vi "EXO1_DatabaseWrite_valves.vi"() -> ()   [LabVIEW 2012]
uses:
  <vilib>/addons/database/Connection.llb/DB Tools Open Connec (Path).vi
  <vilib>/addons/database/NI_Database_API.lvlib
panel:
  in  "V-15":bool
  in  "V-14":bool
  in  "V-13":bool
  in  "V-12":bool
  in  "V-11":bool
  in  "V-10":bool
  in  "V-9":bool
  in  "V-8":bool
  in  "V-7":bool
  in  "V-6":bool
  in  "V-5":bool
  in  "V-4":bool
  in  "V-3":bool
  in  "V-2":bool
  in  "V-1":bool
  in  "stop":bool
  out "current time":timestamp
  in  "Table Name (The table that you want to save the data into)":string="EXOvalve"
  # "EXO DatabaseWrite Sub-VI (II)"
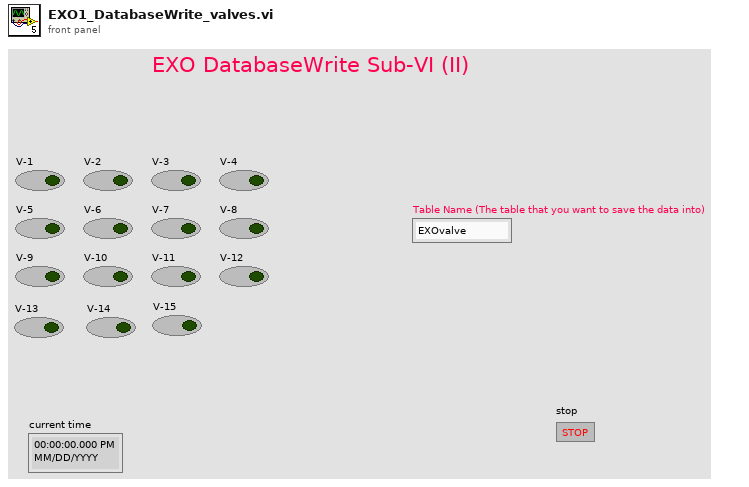
[diagram p1: front panel]
types:
  T1 = typedef "NI_Database_API.lvlib/Conn ObjectReference.ctl" = refnum<k1>
  T2 = cluster{dbl, "date/time string":string, string, string, string, string, string, string, string, string, string, string, string, string, string, string, string}
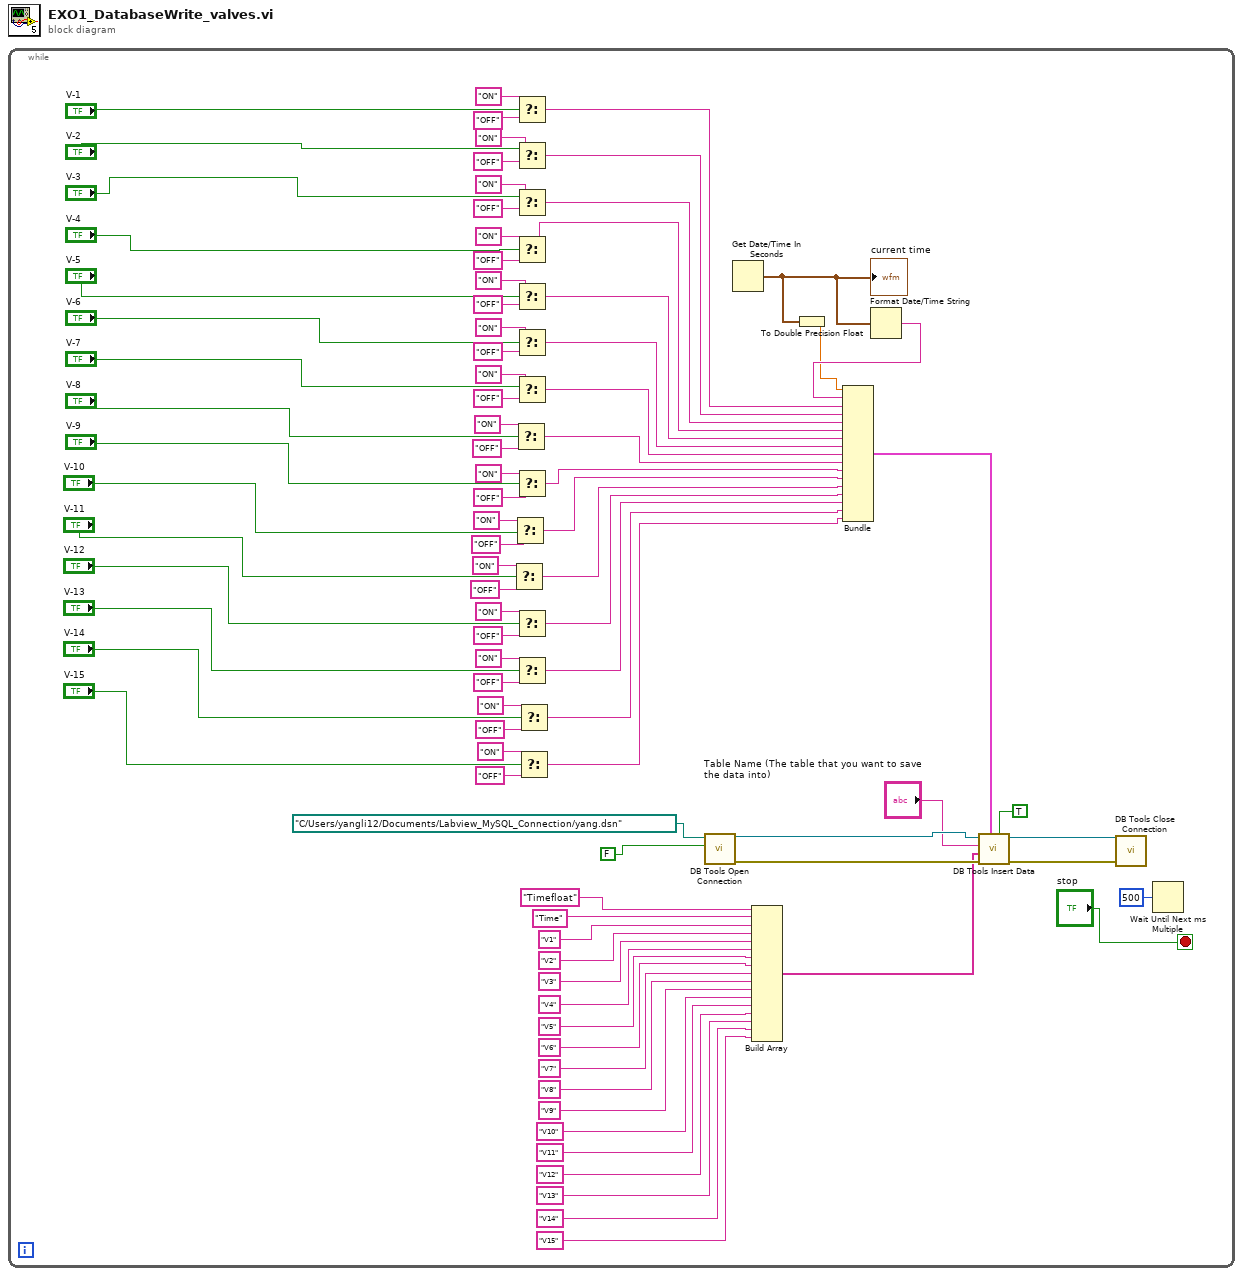
[diagram p0: block diagram]
diagram:
  n1 = while {
    stop <- "stop" stop-if-true
    n2 = Select(t="ON", s="V-11", f="OFF") -> (s? t:f=w22:string)
    n3 = Select(t="ON", s="V-10", f="OFF") -> (s? t:f=w23:string)
    n4 = Select(t="ON", s="V-8", f="OFF") -> (s? t:f=w25:string)
    n5 = Select(t="ON", s="V-1", f="OFF") -> (s? t:f=w60:string)
    n6 = Select(t="ON", s="V-2", f="OFF") -> (s? t:f=w57:string)
    n7 = Select(t="ON", s="V-3", f="OFF") -> (s? t:f=w30:string)
    n8 = Select(t="ON", s="V-4", f="OFF") -> (s? t:f=w29:string)
    n9 = Select(t="ON", s="V-5", f="OFF") -> (s? t:f=w28:string)
    n10 = Select(t="ON", s="V-6", f="OFF") -> (s? t:f=w27:string)
    n11 = Select(t="ON", s="V-7", f="OFF") -> (s? t:f=w26:string)
    n12 = Select(t="ON", s="V-9", f="OFF") -> (s? t:f=w24:string)
    n13 = Select(t="ON", s="V-12", f="OFF") -> (s? t:f=w21:string)
    n14 = Select(t="ON", s="V-13", f="OFF") -> (s? t:f=w18:string)
    n15 = Select(t="ON", s="V-14", f="OFF") -> (s? t:f=w17:string)
    n16 = Select(t="ON", s="V-15", f="OFF") -> (s? t:f=w16:string)
    n17 = call-poly <vilib>:"DB Tools Open Connection.vi"("prompt? (F)"=FALSE, "connection information"=path "C:/Users/yangli12/Documents/Labview_MySQL_Connection/yang.dsn") -> ("error out"=w86:errorcluster, "connection reference"=w87:T1)  [unwired: 6 in]
    n18 = Get Date/Time In Seconds() -> (seconds since 1Jan1904=w78:timestamp)
    "current time" <- w78
    n19 = Build Array("Timefloat" ("element"), "Time" ("table"), "V1" ("table"), "V2" ("table"), "V3" ("table"), "V4" ("table"), "V5" ("table"), "V6" ("table"), "V7" ("table"), "V8" ("table"), "V9" ("table"), "V10" ("table"), "V11" ("table"), "V12" ("table"), "V13" ("table"), "V14" ("table"), "V15" ("table")) -> (w81:string[])
    n20 = To Double Precision Float(number=w78) -> (double precision float=w77:dbl)
    n21 = Format Date/Time String(seconds (now)=w78) -> (date/time string=w79:string)  [unwired: 2 in]
    n22 = Bundle(w77, "date/time string"=w79, w60, w57, w30, w29, w28, w27, w26, w25, w24, w23, w22, w21, w18, w17, w16) -> (w85:T2)  [unwired: 1 in]
    n23 = call <vilib>:"DB Tools Insert Data.vi"("create table? (F)"=TRUE, "data"=w85, "error in (no error)"=w86, "columns"=w81, "table"="Table Name (The table that you want to save the data into)", "connection reference"=w87) -> ("error out"=w75:errorcluster, "connection reference out"=w76:T1)  [unwired: 4 in]
    n24 = call <vilib>:"DB Tools Close Connection.vi"("error in (no error)"=w75, "connection reference"=w76) -> ()  [unwired: 5 in, 1 out]
    n25 = Wait Until Next ms Multiple(millisecond multiple=u32 500) -> ()  [unwired: 1 out]
  }
